vi "Populate Attr XML Priv.vi"(0 "DOM Doc In":refnum<k20>, 2 "Data Types Dict":variant, 5 "Parent Node In":refnum<k20>, 7 "Unique ID":string, 11 "error in":errorcluster, 12 "Attribute Names":string[](array[string]), 13 "Attribute Values":variant[](array[variant])) -> (4 "DOM Doc Out":refnum<k20>, 6 "Parent Node Out":refnum<k20>, 15 "error out":errorcluster)   [LabVIEW 2016, in "Tree Manager.lvclass"]
uses:
  Tree Manager.lvclass
  Tree Data/Tree Data.lvclass
  <vilib>/xml/Close Reference(Node).vi
  <vilib>/xml/NI_XML.lvlib
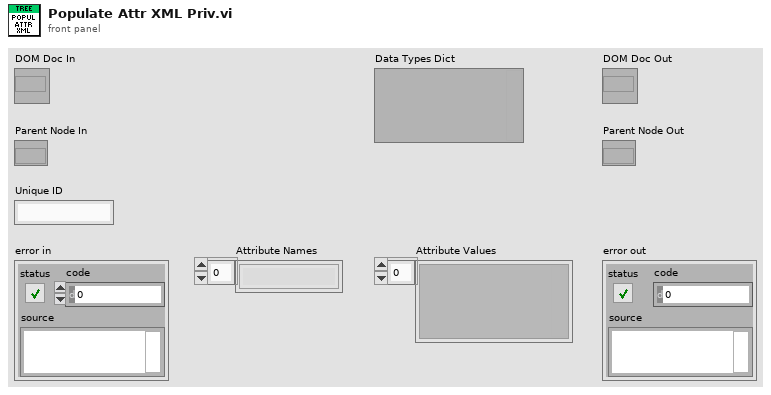
[diagram p1: front panel]
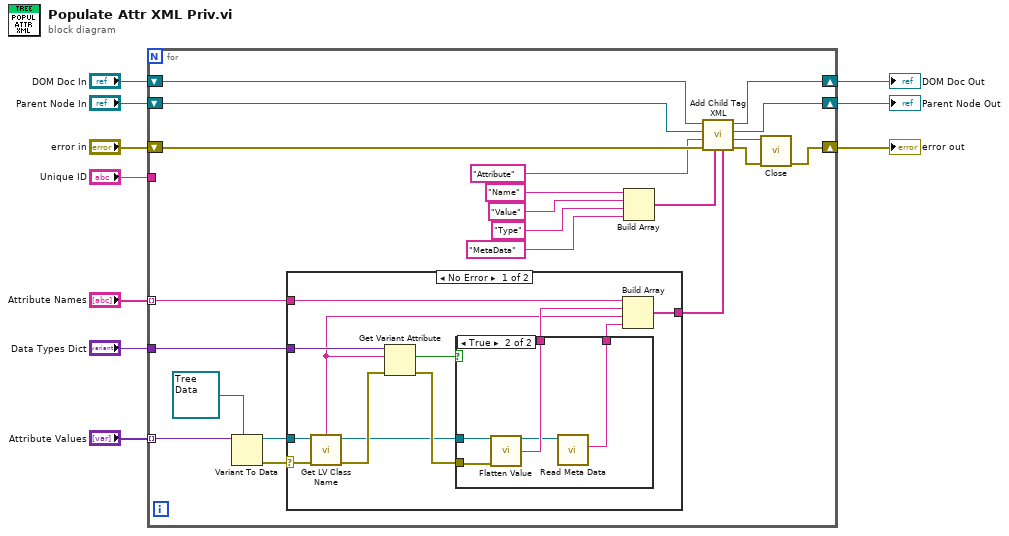
[diagram p0: block diagram]
diagram:
  n1 = for {
    shift-right: [w12] -> w10
    shift-left: "error in" -> [w26]
    tunnel: "Attribute Names" -> [w28] mode=indexing
    tunnel: "Unique ID" -> [_]
    tunnel: "Attribute Values" -> [w31] mode=indexing
    tunnel: "Data Types Dict" -> [w27]
    shift-right: [w24] -> w2
    shift-left: "DOM Doc In" -> [w25]
    shift-right: [w22] -> w1
    shift-left: "Parent Node In" -> [w23]
    n2 = Variant To Data(type=refnum<class "Tree Data.lvclass"> refnum ("Tree Data.lvclass"), Variant=w31) -> (data=w30:refnum<class "Tree Data.lvclass">, error out=w29:errorcluster)  [unwired: 1 in]
    n3 = case shown="No Error" w29 {
      selector: w29 -> [w38 _]
      tunnel: w30 -> [w32 _]
      tunnel: [w40 _] -> w15
      tunnel: w28 -> [w39 _]
      tunnel: w27 -> [w37 _]
      frame No Error {
        n4 = call <vilib>:"Get LV Class Name.vi"("error in (no error)"=w38, "object"=w32) -> ("error out"=w36:errorcluster, "class name"=w33:string)  [unwired: 8 in]
        n5 = Get Variant Attribute(Variant=w37, name=w33, error in=w36) -> (found=w34:bool, error out=w35:errorcluster)  [unwired: 1 in, 2 out]
        n6 = case shown="True" w34 {
          tunnel: [_ w47] -> w42
          tunnel: [_ w46] -> w41
          tunnel: w35 -> [_ w43]
          tunnel: w32 -> [_ w44]
          frame False {
          }
          frame True {
            n7 = call-dynamic "Flatten Value.vi"("Tree Data In"=w44, "Error In"=w43) -> ("Tree Data Out"=w45:refnum<class "Tree Data.lvclass">, "Value"=w47:string)  [unwired: 11 in, 1 out]
            n8 = call "Read Meta Data.vi"("Tree Data In"=w45) -> ("Meta Data"=w46:string)  [unwired: 9 in, 1 out]
          }
        }
        n9 = Build Array(w39, w42, w33, w41) -> (w40:string[])
      }
      frame Error {
      }
    }
    n10 = Build Array("Name" ("Left Cell String"), "Value" ("Left Cell String"), "Type" ("Left Cell String"), "MetaData" ("Left Cell String")) -> (w16:string[])
    n11 = call "Add Child Tag XML.vi"("Values"=w15, "Names"=w16, "Error In"=w26, "Tag Name"="Attribute" ("Left Cell String"), "Parent Node"=w23, "DOM In"=w25) -> ("Error Out"=w13:errorcluster, "Child Node"=w14:refnum<k20>, "Parent Node"=w22:refnum<k20>, "DOM Out"=w24:refnum<k20>)  [unwired: 2 in]
    n12 = call-poly <vilib>:"Close.vi"("error in (no error)"=w13, "node"=w14) -> ("error out"=w12:errorcluster)  [unwired: 7 in]
  }
  "DOM Doc Out" <- w2
  "Parent Node Out" <- w1
  "error out" <- w10
